vi "VISA_Read _to_Number.vi"(6 "Echo Mode":i32, 9 "Command":T1, 11 "Answer Buffer":string) -> (1 "number (I32)":i32, 3 "number (string)":string)   [LabVIEW 2018]
uses:
  MCode_LV_86/Set Parameter.ctl
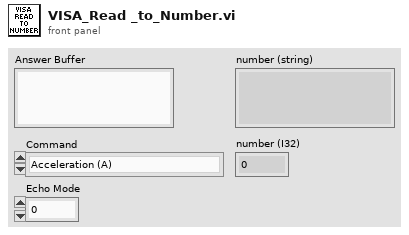
[diagram p1: front panel]
types:
  T1 = typedef "Set Parameter.ctl" = enum16{"Acceleration (A)", "Baud Rate (BD)", "Counter 1 (C1)", "Counter 2 (C2)", "Control C Software Reset (CE)", "Check Sum Enable (CK)", "Clock Mode (CM)", "Clock Mode Ratio (CR)", "Clock Mode Out Step Width (CW)", "Deceleration (D)", "Digital Filtering, Input 1 (D1)", "Digital Filtering, Input 2 (D2)", "Digital Filtering, Input 3 (D3)", "Digital Filtering, Input 4 (D4)", "Digital Filtering, Input 5 (D5)", "Digital Filtering, Input 9 (D9)", "Digital Filtering, Input 10 (D10)", "Digital Filtering, Input 11 (D11)", "Digital Filtering, Input 12 (D12)", "Deadband (DB)", "Decrement Variable (DC)", "Enable/Disable Drive (DE)", "Device Name (DN)", "End Program Execution (E)", "Encoder Function Enable (EE)", "Error Flag (EF)", "Encoder Lines (EL)", "Echo Mode (EM)", "Error Value (ER)", "Escape (ES)", "Execute Program at Address (EX)", "Firmware Version (VR)", "Hold (H)", "Hold Current (HC)", "Hold Current Delay Time (HI)", "Home to Encoder Index (HM)", "Home to Home Switch (HT)", "Increment Variable (IC)", "Initialize Parameters to NVM (IP)", "Input into Variable (IV)", "Jog Enable (JE)", "Limit Stop Mode (LM)", "Move Absolute (MA)", "Move Relative (MR)", "MicroStepping Select (MS)", "Motor Settling Delay Time (MT)", "Moving [Flag] (MV)", "Output 1 (O1)", "Output 2 (O2)", "Output 3 (O3)", "Output 4 (O4)", "Output 9 (O9)", "Output 10 (O10)", "Output 11 (O11)", "Output 12 (O12)", "Output High Byte (9-12) (OH)", "Output Low Byte (1-4) (OL)", "Output Total (1-4 and 9-12) (OT)", "Position (P)", "Position Maintenance (PM)", "Party Mode (PY)", "Register 1 (R1)", "Register 2 (R2)", "Register 3 (R3)", "Register 4 (R4)", "Reset Error(\\03)", "Run Current (RC)", "Stall Factor (SF)", "Slew (SL)", "Stall Mode Set (SM)", "Upgrade Firmware (UG)", "Velocity Initial (VI)", "Velocity Maximum (VM)", "Current1 (I1)", "Current2 (I2)", "Current3 (I3)", "Current4 (I4)", "Current5 (I5)", "Current6 (I6)", "Save (S)"}
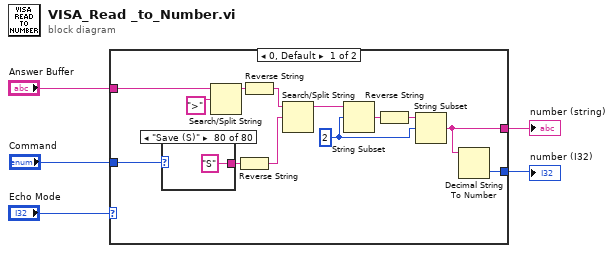
[diagram p0: block diagram]
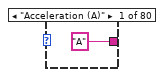
[diagram p2: hidden frame]
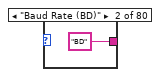
[diagram p3: hidden frame]
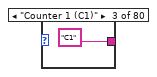
[diagram p4: hidden frame]
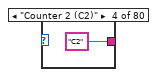
[diagram p5: hidden frame]
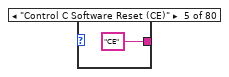
[diagram p6: hidden frame]
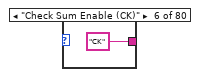
[diagram p7: hidden frame]
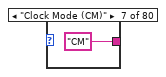
[diagram p8: hidden frame]
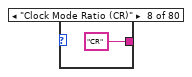
[diagram p9: hidden frame]
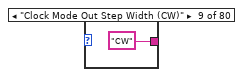
[diagram p10: hidden frame]
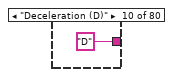
[diagram p11: hidden frame]
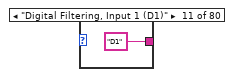
[diagram p12: hidden frame]
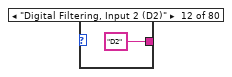
[diagram p13: hidden frame]
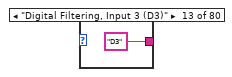
[diagram p14: hidden frame]
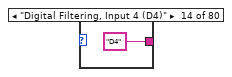
[diagram p15: hidden frame]
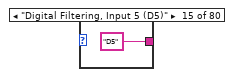
[diagram p16: hidden frame]
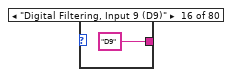
[diagram p17: hidden frame]
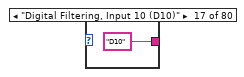
[diagram p18: hidden frame]
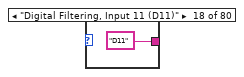
[diagram p19: hidden frame]
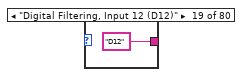
[diagram p20: hidden frame]
diagram:
  n1 = case shown="0, Default" "Echo Mode" {
    tunnel: "Command" -> [w16 _]
    tunnel: [w8 w100] -> w4
    tunnel: [w7 w101] -> w3
    tunnel: "Answer Buffer" -> [w6 w102]
    frame 0, Default {
      w9 = 2
      n2 = case shown="\"Save (S)\"" w16 {
        tunnel: ["A" ("string") "BD" ("string") "C1" ("string") "C2" ("string") "CE" ("string") "CK" ("string") "CM" ("string") "CR" ("string") "CW" ("string") "D" ("string") "D1" ("string") "D2" ("string") "D3" ("string") "D4" ("string") "D5" ("string") "D9" ("string") "D10" ("string") "D11" ("string") "D12" ("string") "DB" ("string") "DC" ("string") "DE" ("string") "DN" ("string") "E" ("string") "EE" ("string") "EF" ("string") "EM" ("string") "ER" ("string") "ES" ("string") "EX" ("string") "VR" ("string") "H" ("string") "HC" ("string") "HI" ("string") "HM" ("string") "HT" ("string") "IC" ("string") "IP" ("string") "IV" ("string") "JE" ("string") "LM" ("string") "MA" ("string") "MR" ("string") "MS" ("string") "MT" ("string") "O1" ("string") "O2" ("string") "O3" ("string") "O4" ("string") "O9" ("string") "O10" ("string") "O11" ("string") "O12" ("string") "OH" ("string") "OL" ("string") "OT" ("string") "P" ("string") "PM" ("string") "PY" ("string") "R1" ("string") "R2" ("string") "R3" ("string") "R4" ("string") "RC" ("string") "SF" ("string") "SL" ("string") "SM" ("string") "UG" ("string") "VI" ("string") "VM" ("string") "EL" ("string") "\u0003" "MV" ("string") "I1" ("string") "I2" ("string") "I3" ("string") "I4" ("string") "I5" ("string") "I6" ("string") "S" ("string")] -> w14
        frame "Acceleration (A)" {
        }
        frame "Baud Rate (BD)" {
        }
        frame "Counter 1 (C1)" {
        }
        frame "Counter 2 (C2)" {
        }
        frame "Control C Software Reset (CE)" {
        }
        frame "Check Sum Enable (CK)" {
        }
        frame "Clock Mode (CM)" {
        }
        frame "Clock Mode Ratio (CR)" {
        }
        frame "Clock Mode Out Step Width (CW)" {
        }
        frame "Deceleration (D)" {
        }
        frame "Digital Filtering, Input 1 (D1)" {
        }
        frame "Digital Filtering, Input 2 (D2)" {
        }
        frame "Digital Filtering, Input 3 (D3)" {
        }
        frame "Digital Filtering, Input 4 (D4)" {
        }
        frame "Digital Filtering, Input 5 (D5)" {
        }
        frame "Digital Filtering, Input 9 (D9)" {
        }
        frame "Digital Filtering, Input 10 (D10)" {
        }
        frame "Digital Filtering, Input 11 (D11)" {
        }
        frame "Digital Filtering, Input 12 (D12)" {
        }
        frame "Deadband (DB)" {
        }
        frame "Decrement Variable (DC)" {
        }
        frame "Enable/Disable Drive (DE)" {
        }
        frame "Device Name (DN)" {
        }
        frame "End Program Execution (E)" {
        }
        frame "Encoder Function Enable (EE)" {
        }
        frame "Error Flag (EF)" {
        }
        frame "Echo Mode (EM)" {
        }
        frame "Error Value (ER)" {
        }
        frame "Escape (ES)" {
        }
        frame "Execute Program at Address (EX)" {
        }
        frame "Firmware Version (VR)" {
        }
        frame "Hold (H)" {
        }
        frame "Hold Current (HC)" {
        }
        frame "Hold Current Delay Time (HI)" {
        }
        frame "Home to Encoder Index (HM)" {
        }
        frame "Home to Home Switch (HT)" {
        }
        frame "Increment Variable (IC)" {
        }
        frame "Initialize Parameters to NVM (IP)" {
        }
        frame "Input into Variable (IV)" {
        }
        frame "Jog Enable (JE)" {
        }
        frame "Limit Stop Mode (LM)" {
        }
        frame "Move Absolute (MA)" {
        }
        frame "Move Relative (MR)" {
        }
        frame "MicroStepping Select (MS)" {
        }
        frame "Motor Settling Delay Time (MT)" {
        }
        frame "Output 1 (O1)" {
        }
        frame "Output 2 (O2)" {
        }
        frame "Output 3 (O3)" {
        }
        frame "Output 4 (O4)" {
        }
        frame "Output 9 (O9)" {
        }
        frame "Output 10 (O10)" {
        }
        frame "Output 11 (O11)" {
        }
        frame "Output 12 (O12)" {
        }
        frame "Output High Byte (9-12) (OH)" {
        }
        frame "Output Low Byte (1-4) (OL)" {
        }
        frame "Output Total (1-4 and 9-12) (OT)" {
        }
        frame "Position (P)" {
        }
        frame "Position Maintenance (PM)" {
        }
        frame "Party Mode (PY)" {
        }
        frame "Register 1 (R1)" {
        }
        frame "Register 2 (R2)" {
        }
        frame "Register 3 (R3)" {
        }
        frame "Register 4 (R4)" {
        }
        frame "Run Current (RC)" {
        }
        frame "Stall Factor (SF)" {
        }
        frame "Slew (SL)" {
        }
        frame "Stall Mode Set (SM)" {
        }
        frame "Upgrade Firmware (UG)" {
        }
        frame "Velocity Initial (VI)" {
        }
        frame "Velocity Maximum (VM)" {
        }
        frame "Encoder Lines (EL)" {
        }
        frame "Reset Error(\\03)" {
        }
        frame "Moving [Flag] (MV)" {
        }
        frame "Current1 (I1)" {
        }
        frame "Current2 (I2)" {
        }
        frame "Current3 (I3)" {
        }
        frame "Current4 (I4)" {
        }
        frame "Current5 (I5)" {
        }
        frame "Current6 (I6)" {
        }
        frame "Save (S)" {
        }
      }
      n3 = Search/Split String(string=w6, search string/char (-)=">") -> (substring before match=w17:string)  [unwired: 1 in, 2 out]
      n4 = Reverse String(1:w14) -> (0:w13:string)
      n5 = Reverse String(1:w17) -> (0:w15:string)
      n6 = Search/Split String(string=w15, search string/char (-)=w13) -> (substring before match=w12:string)  [unwired: 1 in, 2 out]
      n7 = String Subset(string=w12, offset (0)=w9) -> (substring=w11:string)  [unwired: 1 in]
      n8 = Reverse String(1:w11) -> (0:w10:string)
      n9 = String Subset(string=w10, offset (0)=w9) -> (substring=w8:string)  [unwired: 1 in]
      n10 = Decimal String To Number(string=w8) -> (number=w7:i32)  [unwired: 2 in, 1 out]
    }
    frame 2 {
      n11 = Search/Split String(string=w102, search string/char (-)="\r\n") -> (substring before match=w100:string)  [unwired: 1 in, 2 out]
      n12 = Decimal String To Number(string=w100) -> (number=w101:i32)  [unwired: 2 in, 1 out]
    }
  }
  "number (string)" <- w4
  "number (I32)" <- w3
